vi "Teleop.vi"(9 "Match Info":T1={"Autonomous Elapsed Seconds"=0.0, "TeleOp Elapsed Seconds"=0.0, "Disabled Elapsed Seconds"=0.0, "Visited Autonomous"=FALSE, "Visited TeleOp"=FALSE, "Visited Disabled"=FALSE, "Autonomous Settings"={"Autonomous Style"=enum."Independent", "VI Refnum"=refnum}}, 11 "Call Context":T2) -> ()   [LabVIEW 2013]
doc: "This VI is called for each TeleOp packet received from the DS where the robot is not disabled. It is often used to read from the joysticks and update I/O or to update setpoints for timed control loops. It should complete and return within 20 milliseconds or it may miss DS packets."
uses:
  <vilib>/Rock Robotics/WPI/DriverStation/WPI_DriverStationDerivedRobotMode.ctl
  <vilib>/Rock Robotics/WPI/DriverStation/WPI_DriverStationMatch Info.ctl
  Robot Global Data.vi
  <vilib>/addons/control/pid/pid.llb/PID (DBL).vi
  <vilib>/Rock Robotics/WPI/RobotDrive/WPI_RobotDriveGetSetRefNum.vi
  <vilib>/addons/control/pid/NI_PID_pid.lvlib
panel:
  in  "reinitialize? (F)":bool
  out "Encoder Rate":cluster{"Rate":dbl, "Rate":dbl}
  in  "D":dbl
  in  "I":dbl
  in  "P":dbl
  out "error out":errorcluster
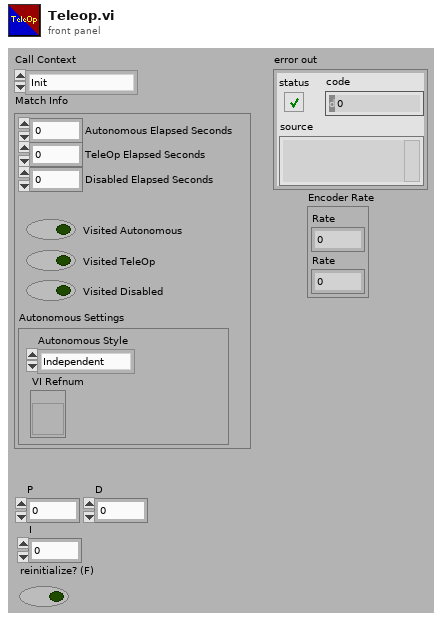
[diagram p1: front panel]
types:
  T1 = typedef "WPI_DriverStationMatch Info.ctl" = cluster{"Autonomous Elapsed Seconds":dbl, "TeleOp Elapsed Seconds":dbl, "Disabled Elapsed Seconds":dbl, "Visited Autonomous":bool, "Visited TeleOp":bool, "Visited Disabled":bool, "Autonomous Settings":cluster{"Autonomous Style":enum16{"Iterative", "Independent"}, "VI Refnum":refnum<vi>}}
  T2 = typedef "WPI_DriverStationDerivedRobotMode.ctl" = enum16{"Init", "Execute", "Stop"}
  T3 = typedef "WPI_RobotDriveDevRef.ctl" = cluster{"DevStatus":errorcluster, "Motors[]":T4[], "Square Inputs":bool, "Max Output":dbl, "Isochronous":bool}
  T4 = typedef "WPI_MotorControlDeviceRef.ctl" = cluster{"DeviceStatus":errorcluster, "Type":enum16{"PWM", "CAN"}, "PWM":cluster{"Digital Module":T5, "PWM Channel":T6, "DeadBand":T7}, "CAN":cluster{"Device Number":u8, "Control Mode":T8, "Semaphore":T9, "Max Vout":dbl}, "Invert":bool, "TransformRef":T10, "InvTransformRef":T10}
  T5 = typedef "FPGA_TypedefDigitalModule.ctl" = enum16{"Digital Module 1", "Digital Module 2"}
  T6 = typedef "FPGA_DIOPWMChannel.ctl" = enum8{"PWM 1", "PWM 2", "PWM 3", "PWM 4", "PWM 5", "PWM 6", "PWM 7", "PWM 8", "PWM 9", "PWM 10", "Invalid"}
  T7 = typedef "WPI_PWMDeadband.ctl" = cluster{"Name":string, "maxPositivePwm":i32, "minPositivePwm":i32, "centerPwm":i32, "maxNegativePwm":i32, "minNegativePwm":i32, "angularRange":u16}
  T8 = typedef "WPI_CANJaguar_ControlMode.ctl" = enum8{"Percent VBus", "Current", "Speed", "Position", "Voltage"}
  T9 = typedef "Semaphore RefNum" = refnum<k1>
  T10 = typedef "WPI_PWMTransform_ConPane.ctl" = refnum<vi>
  T11 = typedef "WPI_EncoderDevRef.ctl" = cluster{"DevStatus":errorcluster, "EncoderIndex":T12, "CounterIndex":T13, "DistancePerCount":dbl, "Decoding Type":T14}
  T12 = typedef "FPGA_EncoderIdx.ctl" = enum8{"Enc 0", "Enc 1", "Enc 2", "Enc 3", "Invalid"}
  T13 = typedef "FPGA_CounterCtrSystemIndex.ctl" = enum8{"Ctr 0", "Ctr 1", "Ctr 2", "Ctr 3", "Ctr 4", "Ctr 5", "Ctr 6", "Ctr 7", "Invalid"}
  T14 = typedef "WPI_EncoderType.ctl" = enum16{"1x", "2x", "4x"}
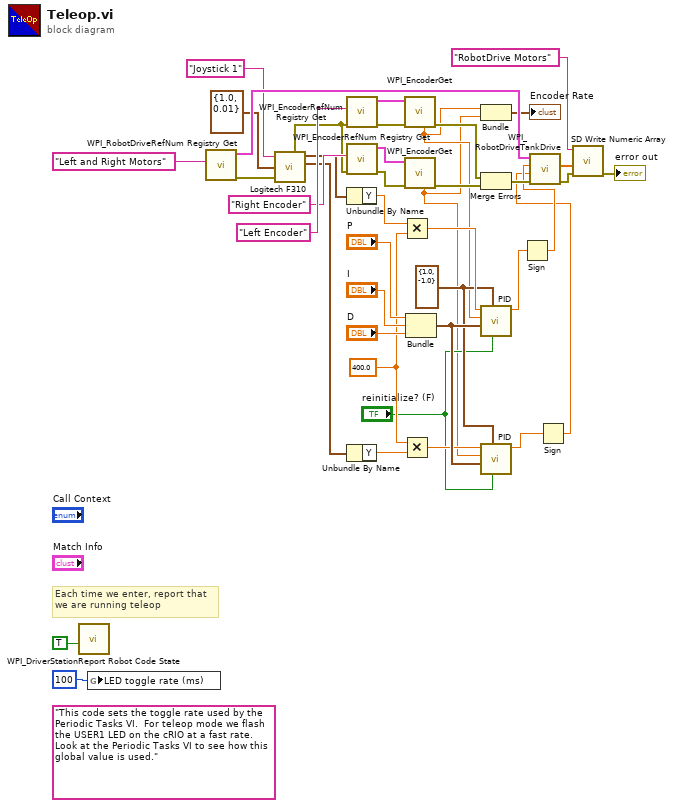
[diagram p0: block diagram]
diagram:
  w15 = cluster{"output high":dbl, "output low":dbl} {"output high"=1.0, "output low"=-1.0} ("output range")
  w16 = 400.0 ("x")
  (unwired) "This code sets the toggle rate used by the Periodic Tasks VI.  For teleop mode we flash the USER1 LED on the cRIO at a fast rate.  Look at the Periodic Tasks VI to see how this global value is used."
  # "Each time we enter, report that\nwe are running teleop"
  n1 = call <vilib>:"WPI_DriverStationReport Robot Code State.vi"("TeleOp"=TRUE ("Autonomous")) -> ()  [unwired: 10 in, 1 out]
  n2 = global write "Robot Global Data.vi" "LED toggle rate (ms)"(u32 100 ("LED ms toggle rate")) -> ()
  n3 = call <vilib>:"WPI_RobotDriveRefNum Registry Get.vi"("refnum name"="Left and Right Motors") -> ("error out"=w12:errorcluster, "RobotDriveDevRef"=w38:T3)  [unwired: 9 in]
  n4 = call "Logitech F310.vi"("error in (no error)"=w12, "Deadzone Scale Cluster"=cluster{"Scale":dbl, "Deadzone":dbl} {"Scale"=1.0, "Deadzone"=0.01}, "refnum name"="Joystick 1") -> ("Right Stick"=w7:cluster{"X":dbl, "Y":dbl}, "error out"=w9:errorcluster, "Left Stick"=w8:cluster{"X":dbl, "Y":dbl})  [unwired: 3 out]
  n5 = call <vilib>:"WPI_EncoderRefNum Registry Get.vi"("error in (no error)"=w9, "refnum name"="Left Encoder") -> ("error out"=w26:errorcluster, "EncoderDevRef"=w25:T11)  [unwired: 8 in]
  n6 = call <vilib>:"WPI_EncoderRefNum Registry Get.vi"("error in (no error)"=w9, "refnum name"="Right Encoder") -> ("error out"=w24:errorcluster, "EncoderDevRef"=w23:T11)  [unwired: 8 in]
  n7 = Unbundle By Name(w8) -> ("Y"=w30:dbl)
  n8 = Unbundle By Name(w7) -> ("Y"=w29:dbl)
  n9 = Multiply(x=w30, y=w16) -> (x*y=w18:dbl)
  n10 = Multiply(x=w16, y=w29) -> (x*y=w17:dbl)
  n11 = call <vilib>:"WPI_EncoderGet.vi"("error in (no error)"=w26, "EncoderDevRef"=w25) -> ("error out"=w20:errorcluster, "Rate"=w6:dbl)  [unwired: 4 in, 4 out]
  n12 = call <vilib>:"WPI_EncoderGet.vi"("error in (no error)"=w24, "EncoderDevRef"=w23) -> ("error out"=w21:errorcluster, "Rate"=w5:dbl)  [unwired: 4 in, 4 out]
  n13 = Bundle("P"="P", "I"="I", "D"="D") -> (w28:cluster{"P":dbl, "I":dbl, "D":dbl})  [unwired: 1 in]
  n14 = Bundle("Rate"=w6, "Rate"=w5) -> (→"Encoder Rate":cluster{"Rate":dbl, "Rate":dbl})  [unwired: 1 in]
  n15 = Merge Errors(w20, w21) -> (w19:errorcluster)
  n16 = call-poly <vilib>:"PID.vi"("reinitialize? (F)"="reinitialize? (F)", "output range"=w15, "PID gains"=w28, "process variable"=w6, "setpoint"=w18) -> ("output"=w4:dbl)  [unwired: 5 in, 1 out]
  n17 = call-poly <vilib>:"PID.vi"("reinitialize? (F)"="reinitialize? (F)", "output range"=w15, "PID gains"=w28, "process variable"=w5, "setpoint"=w17) -> ("output"=w2:dbl)  [unwired: 5 in, 1 out]
  n18 = Sign(1:w4) -> (0:w3:dbl)
  n19 = Sign(1:w2) -> (0:w1:dbl)
  n20 = call <vilib>:"WPI_RobotDriveTankDrive.vi"("error in (no error)"=w19, "Right axis value"=w1, "Left axis value"=w3, "RobotDriveDevRef"=w38) -> ("error out"=w36:errorcluster, "Motor Values"=w37:dbl[])  [unwired: 5 in, 1 out]
  n21 = call <vilib>:"SD Write Numeric Array.vi"("error in"=w36, "Numeric Array"=w37, "Name"="RobotDrive Motors") -> ("error out"=→"error out":errorcluster)  [unwired: 7 in, 1 out]
